vi "MB Slave Init (poly).vi"(5 "error in":errorcluster) -> (14 "Holding Registers":u16[](array[numeric]), 15 "Coils":bool[](array[boolean]), 19 "error out":errorcluster)   [LabVIEW 2011]
doc: "You must use this VI to initialize two 65536 U16 arrays (for registers) and two 65536 Boolean arrays (for coils and discrete inputs)."
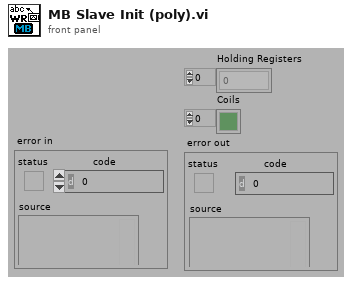
[diagram p1: front panel]
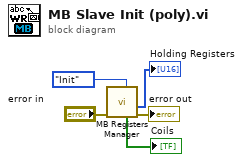
[diagram p0: block diagram]
diagram:
  n1 = call "MB Registers Manager.vi"("Function"=enum16{"Init", "Read", "Write", "Read All"}."Init", "error in (no error)"="error in") -> ("error out"=→"error out":errorcluster, "Words out"=→"Holding Registers":u16[], "Bits out"=→"Coils":bool[])  [unwired: 5 in, 2 out]
